vi "Barcode_Generator.vi"() -> ()   [LabVIEW 2021]
panel:
  in  "Print Mode":bool
  in  "Path to PNG File":path
  out "Final CMD":string
  in  "CMD Right":string
  in  "CMD Left":string
  in  "Input Barcode":string
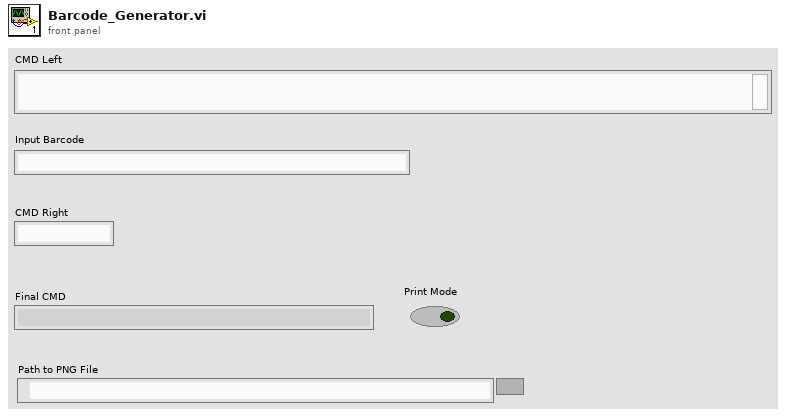
[diagram p1: front panel]
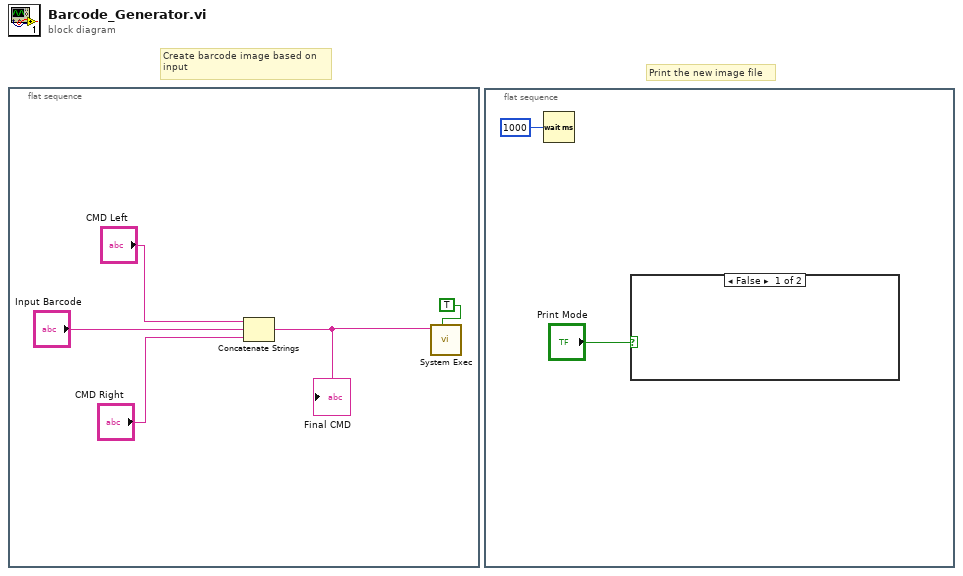
[diagram p0: block diagram]
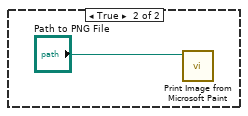
[diagram p2: hidden frame]
diagram:
  # "Print the new image file"
  # "Create barcode image based on\ninput"
  n1 = flat-sequence {
    frame #0 {
      n2 = Concatenate Strings("CMD Left", "Input Barcode", "CMD Right") -> (w5:string)
      "Final CMD" <- w5
      n3 = call <vilib>:"System Exec.vi"("wait until completion? (T)"=TRUE, "command line"=w5) -> ()  [unwired: 6 in, 4 out]
    }
  }
  n4 = flat-sequence {
    frame #0 {
      n5 = Wait (ms)(milliseconds to wait=u32 1000) -> ()  [unwired: 1 out]
      n6 = case shown="False" "Print Mode" {
        frame False {
        }
        frame True {
          n7 = call "Print Image from Microsoft Paint.vi"("Path to PNG File"="Path to PNG File") -> ()  [unwired: 10 in, 1 out]
        }
      }
    }
  }
